vi "Configure Modem.vi"(8 "error in (no error)":errorcluster, 11 "Data Cluster":T1={"Data Display"="", "FP Control Refs"={"Connect to Station Ref"=refnum, "Download Ref"=refnum, "Exit Button Ref"=refnum, "Start Date Refnum"=refnum, "End Date Refnum"=refnum, "Path"=refnum, "COM Port"="", "IP or Phone Ref"=refnum, "TCPIP ID"=refnum, "Reboot Refnum"=refnum, "Datafile Refnum"=refnum}, "FP Indicator Refs"={"Connected Refnum"=refnum, "Data Display Ref"=refnum, "Station ID Ref"=refnum}, "User Events"={"Stop"=refnum, "Update Display"=refnum}, "Message Queues"={"UI"=refnum, "ACQUISITION"=refnum, "PROCESSING"=refnum, "LOGGING"=refnum}, "IS IP?"=FALSE, "Downloading?"=FALSE, "DCP Version"=enum."XPert2", "Processing Loop State"=enum."Get Station  ID", "Username"=refnum, "Password"=refnum}) -> (0 "error out":errorcluster, 3 "Data Cluster out":T1={"Data Display"="", "FP Control Refs"={"Connect to Station Ref"=refnum, "Download Ref"=refnum, "Exit Button Ref"=refnum, "Start Date Refnum"=refnum, "End Date Refnum"=refnum, "Path"=refnum, "COM Port"="", "IP or Phone Ref"=refnum, "TCPIP ID"=refnum, "Reboot Refnum"=refnum, "Datafile Refnum"=refnum}, "FP Indicator Refs"={"Connected Refnum"=refnum, "Data Display Ref"=refnum, "Station ID Ref"=refnum}, "User Events"={"Stop"=refnum, "Update Display"=refnum}, "Message Queues"={"UI"=refnum, "ACQUISITION"=refnum, "PROCESSING"=refnum, "LOGGING"=refnum}, "IS IP?"=FALSE, "Downloading?"=FALSE, "DCP Version"=enum."XPert2", "Processing Loop State"=enum."Get Station  ID", "Username"=refnum, "Password"=refnum})   [LabVIEW 2018]
uses:
  controls/GLDL UI Data.ctl
  controls/Disconnect Control.ctl
  controls/Download Control.ctl
  controls/Exit Control.ctl
  controls/Date Control.ctl
  controls/IP Phone Number Control.ctl
  controls/Reboot Control.ctl
  controls/Connected Indicator.ctl
  controls/Output Indicator.ctl
  controls/Station ID Indicator.ctl
  Message Queue/All Message Queues.ctl
  Message Queue/Message Cluster.ctl
  controls/Processing Loop State.ctl
  <vilib>/Instr/_visa.llb/VISA Configure Serial Port (Instr).vi
  Message Queue/GLDL Message Queue.lvlib
types:
  T1 = typedef "GLDL UI Data.ctl" = cluster{"Data Display":string, "FP Control Refs":cluster{"Connect to Station Ref":refnum<vi>, "Download Ref":refnum<vi>, "Exit Button Ref":refnum<vi>, "Start Date Refnum":refnum<vi>, "End Date Refnum":refnum<vi>, "Path":refnum<vi>, "COM Port":refnum<visa-resource-name>, "IP or Phone Ref":refnum<vi>, "TCPIP ID":refnum<k5>, "Reboot Refnum":refnum<vi>, "Datafile Refnum":refnum<file>}, "FP Indicator Refs":cluster{"Connected Refnum":refnum<vi>, "Data Display Ref":refnum<vi>, "Station ID Ref":refnum<vi>}, "User Events":cluster{"Stop":refnum<user-event>, "Update Display":refnum<user-event>}, "Message Queues":T2, "IS IP?":bool, "Downloading?":bool, "DCP Version":enum16{"XPert", "XPert2"}, "Processing Loop State":T3, "Username":refnum<vi>, "Password":refnum<vi>}
  T2 = typedef "GLDL Message Queue.lvlib/All Message Queues.ctl" = cluster{"UI":refnum<queue>, "ACQUISITION":refnum<queue>, "PROCESSING":refnum<queue>, "LOGGING":refnum<queue>}
  T3 = typedef "Processing Loop State.ctl" = enum16{"Get Station  ID", "Change Directory SD Card", "Change Directory Storage Card", "Downloading", "Idle in DL Directory"}
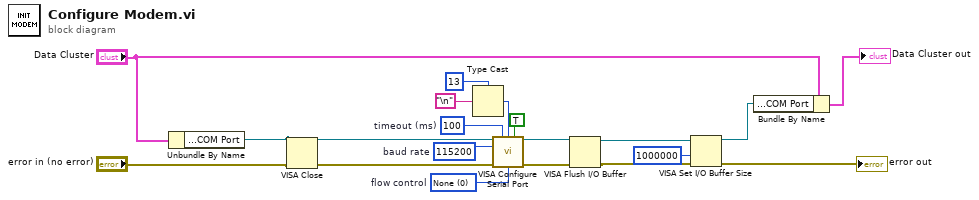
[diagram p0: block diagram]
diagram:
  w19 = u16 0 items=["None", "XON/XOFF", "RTS/CTS", "XON/XOFF & RTS/CTS", "DTR/DSR", "XON/XOFF & DTR/DSR"]  # flow control
  w8 = u32 115200  # baud rate
  w18 = u32 100  # timeout (ms)
  n1 = Unbundle By Name("Data Cluster") -> ("FP Control Refs.COM Port"=w15:refnum<visa-resource-name>)
  n2 = VISA Close(VISA resource name=w15, error in (no error)="error in (no error)") -> (error out=w13:errorcluster)
  n3 = Type Cast(type=u8 13 ("termination char\n(0xA = '\\n' = LF)"), x="\n") -> (*(type *) &x=w10:u8)
  n4 = call-poly "VISA Configure Serial Port"("VISA resource name"=w15, "timeout (10sec)"=w18, "termination char\n(0xA = '\\n' = LF)"=w10, "Enable Termination\nChar (T)"=TRUE ("Enable Termination\nChar (T)"), "baud rate (9600)"=w8, "error in (no error)"=w13, "flow control (0:none)"=w19) -> ("VISA resource name out"=w2:refnum<visa-resource-name>, "error out"=w4:errorcluster)  [unwired: 7 in]
  n5 = VISA Flush I/O Buffer(VISA resource name=w2, error in (no error)=w4) -> (VISA resource name out=w1:refnum<visa-resource-name>, error out=w3:errorcluster)  [unwired: 1 in]
  n6 = VISA Set I/O Buffer Size(VISA resource name=w1, size (4096)=u32 1000000, error in (no error)=w3) -> (VISA resource name out=w7:refnum<visa-resource-name>, error out=→"error out":errorcluster)  [unwired: 1 in]
  n7 = Bundle By Name(cluster="Data Cluster", "FP Control Refs.COM Port"=w7) -> (→"Data Cluster out":T1)
